vi "Configure Reference Levels [WM] Core.vi"(0 "IVI_Scope in":refnum<class "IVI_Scope.lvclass">, 5 "low reference (10.0%)":dbl=10.0 format="%.3f", 7 "mid reference (50.0%)":dbl=50.0 format="%.3f", 9 "high reference (90.0%)":dbl=90.0 format="%.3f", 11 "error in (no error)":errorcluster) -> (4 "IVI_Scope out":refnum<class "IVI_Scope.lvclass">, 15 "error out":errorcluster)   [LabVIEW 2016, in "IVI_Scope.lvlib" / "IVI_Scope.lvclass"]
doc: "This VI configures the reference levels for waveform measurements. \n\nYou must call this VI before you call the IviScope Read Waveform Measurement [WM] or IviScope Fetch Waveform Measurement [WM] to take a rise time, fall time, width negative, width positive, duty cycle negative, duty cycle positive, preshoot, or overshoot measurement.\n\nNotes:\n\n(1) This VI is part of the IviScopeWaveformMeasurement [WM] extension group."
uses:
  IVI_Scope.lvclass
  IVI_Scope.lvclass/IVI_Scope.ctl
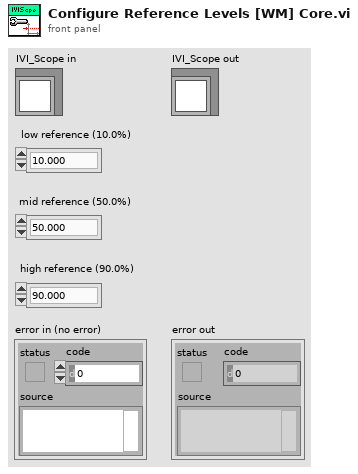
[diagram p1: front panel]
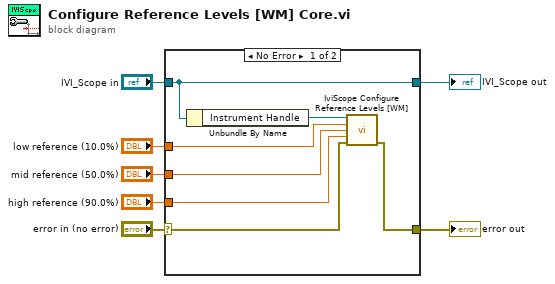
[diagram p0: block diagram]
diagram:
  n1 = case shown="No Error" "error in (no error)" {
    selector: "error in (no error)" -> [w12 w16]
    tunnel: [w11 w16] -> w6
    tunnel: [w14 w15] -> w4
    tunnel: "IVI_Scope in" -> [w14 w15]
    tunnel: "low reference (10.0%)" -> [w10 _]
    tunnel: "mid reference (50.0%)" -> [w9 _]
    tunnel: "high reference (90.0%)" -> [w8 _]
    frame No Error {
      n2 = Unbundle By Name(w14) -> ("Instrument Handle"=w13:refnum<k15>)
      n3 = call <vilib>:"IviScope Configure Reference Levels [WM].vi"("instrument handle"=w13, "low reference (10.0%)"=w10, "mid reference (50.0%)"=w9, "high reference (90.0%)"=w8, "error in (no error)"=w12) -> ("error out"=w11:errorcluster)  [unwired: 9 in, 1 out]
    }
    frame Error {
    }
  }
  "error out" <- w6
  "IVI_Scope out" <- w4
